vi "myRIO v1.0 Write AO.vi"(7 "Scale Constants Array":T1, 8 "error in (no error)":errorcluster, 9 "dbl Scaled Value List":dbl[](array[numeric]), 10 "Channel List":T5, 11 "myRIO Ref In":T3) -> (0 "error out":errorcluster, 3 "myRIO Ref Out":T3)   [LabVIEW 2021]
uses:
  <vilib>/myRIO/Common/Instrument Driver Framework/myRIO v1.0/AO/typedefs/AO Channels List.ctl
  <vilib>/myRIO/Common/Instrument Driver Framework/myRIO v1.0/AO/typedefs/AO Channels Enum.ctl
  <vilib>/myRIO/Common/Instrument Driver Framework/Utilities/typedefs/myRIO v1.0 Reference.ctl
  <vilib>/myRIO/Common/Instrument Driver Framework/Utilities/typedefs/Generic FPGA Reference.ctl
  <vilib>/myRIO/Common/Instrument Driver Framework/Utilities/typedefs/Analog Scaling Constants List.ctl
  <vilib>/myRIO/Common/Instrument Driver Framework/Utilities/typedefs/Analog Scaling Constants.ctl
  <vilib>/myRIO/Common/Instrument Driver Framework/myRIO v1.0/AO/typedefs/AO Channels FPGA Reference.ctl
  <vilib>/rvi/errors/niLvFpgaAdjustHostInterfaceError.vi
  <vilib>/rvi/interface/nirviReadWriteControl/nirviReadWriteControl.xnode
  <vilib>/rvi/interface/Simulation/niFpgaSimulationCallBeginRW.vi
  NiFpgaLv.dll
panel:
  # "This VI write one analog value to a user specified analog output channel on the myRIO v1.0 hardware. The value is input as a dbl value and scaled to a u16 for input to the FPGA based on the specifications of the DAC. Please see Block Diagram for details."
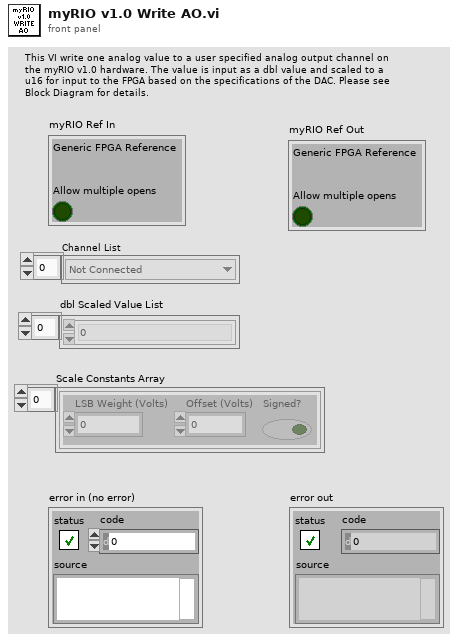
[diagram p1: front panel]
types:
  T1 = typedef "Analog Scaling Constants List.ctl" = T2[]
  T2 = typedef "Analog Scaling Constants.ctl" = cluster{"LSB Weight (Volts)":dbl, "Offset (Volts)":dbl, "Signed?":bool}
  T3 = typedef "myRIO v1.0 Reference.ctl" = cluster{"Generic FPGA Reference":T4, "Allow multiple opens":bool}
  T4 = typedef "Generic FPGA Reference.ctl" = refnum<k20>
  T5 = typedef "AO Channels List.ctl" = T6[]
  T6 = typedef "AO Channels Enum.ctl" = enum16{"Not Connected", "AudioOut/Left", "AudioOut/Right", "C/AO0", "C/AO1", "A/AO0", "A/AO1", "B/AO0", "B/AO1"}
  T7 = typedef "AO Channels FPGA Reference.ctl" = refnum<k20>
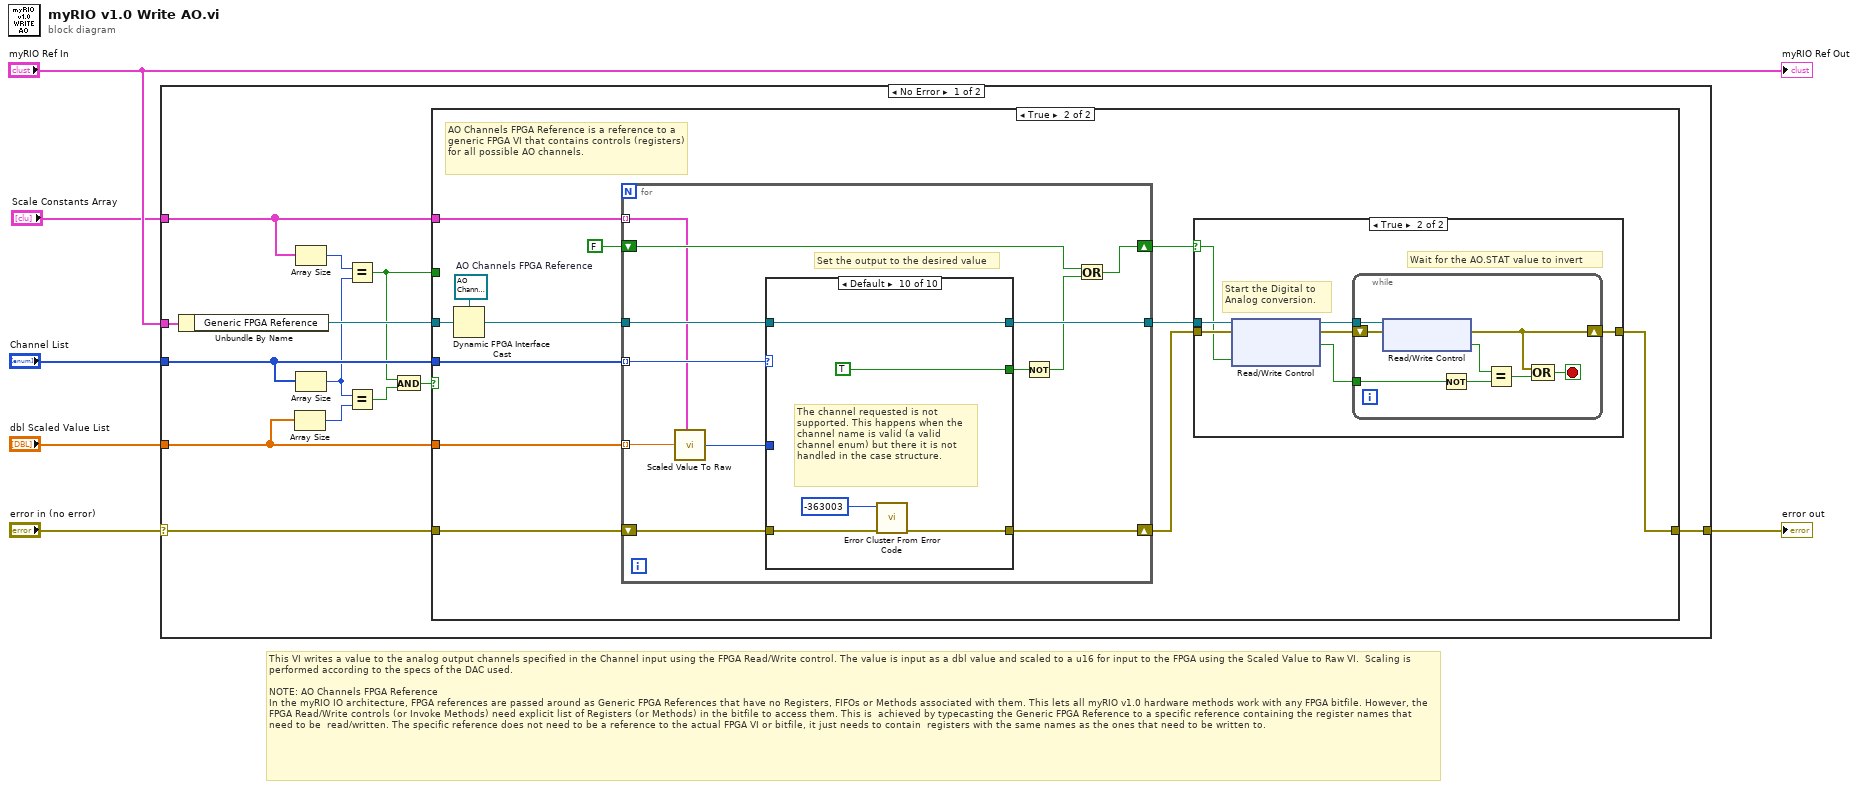
[diagram p0: block diagram]
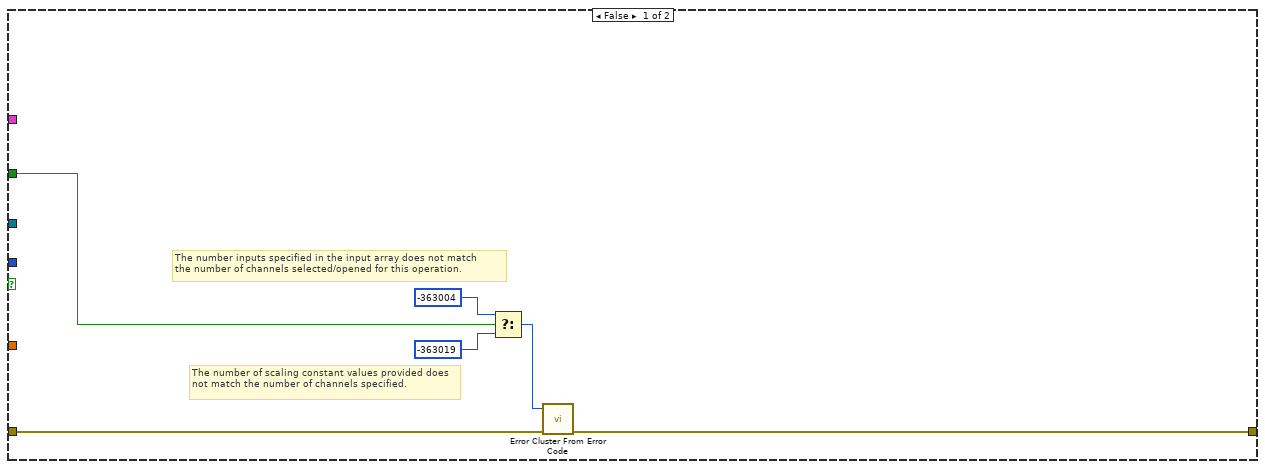
[diagram p2: hidden frame]
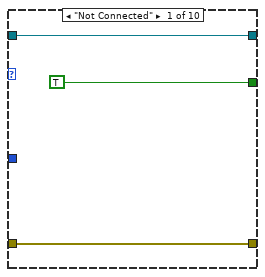
[diagram p4: hidden frame]
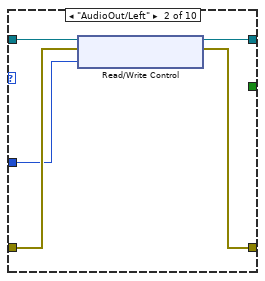
[diagram p5: hidden frame]
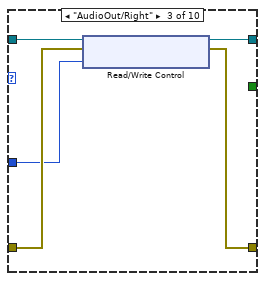
[diagram p6: hidden frame]
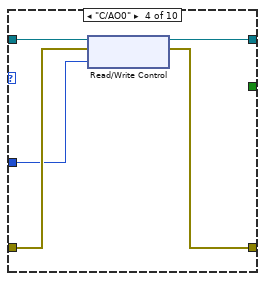
[diagram p7: hidden frame]
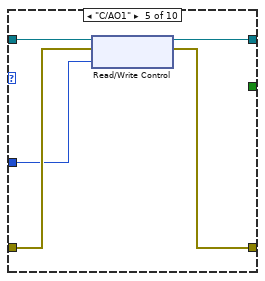
[diagram p8: hidden frame]
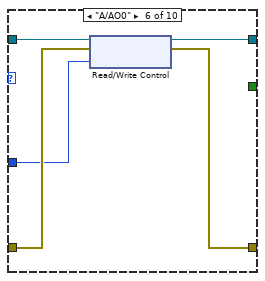
[diagram p9: hidden frame]
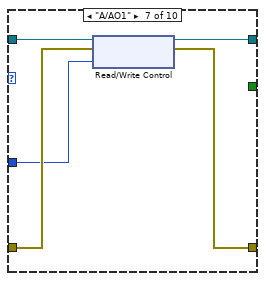
[diagram p10: hidden frame]
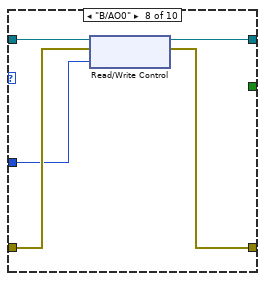
[diagram p11: hidden frame]
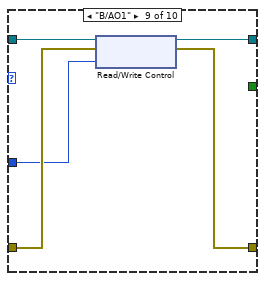
[diagram p12: hidden frame]
diagram:
  # "This VI writes a value to the analog output channels specified in the Channel input using the FPGA Read/Write control. The value is input as a dbl value and scaled to a u16 for input to the FPGA using the Scaled Value to Raw VI.  Scaling is performed according to the specs of the DAC used.\n\nNOTE: AO Channels FPGA Reference\nIn the myRIO IO architecture, FPGA references are passed around as Generic FPGA References that have no Registers, FIFOs or Methods associated with them. This lets all myRIO v1.0 hardware methods work with any FPGA bitfile. However, the  FPGA Read/Write controls (or Invoke Methods) need explicit list of Registers (or Methods) in the bitfile to access them. This is  achieved by typecasting the Generic FPGA Reference to a specific reference containing the register names that need to be  read/written. The specific reference does not need to be a reference to the actual FPGA VI or bitfile, it just needs to contain  registers with the same names as the ones that need to be written to."
  n1 = case shown="No Error" "error in (no error)" {
    selector: "error in (no error)" -> [w15 w114]
    tunnel: [w19 w114] -> w6
    tunnel: "Channel List" -> [w18 _]
    tunnel: "dbl Scaled Value List" -> [w17 _]
    tunnel: "myRIO Ref In" -> [w14 _]
    tunnel: "Scale Constants Array" -> [w12 _]
    frame No Error {
      n2 = Unbundle By Name(w14) -> ("Generic FPGA Reference"=w13:T4)
      n3 = Array Size(array=w17) -> (size(s)=w16:i32)
      n4 = Array Size(array=w12) -> (size(s)=w11:i32)
      n5 = Array Size(array=w18) -> (size(s)=w10:i32)
      n6 = Equal?(x=w11, y=w10) -> (x = y?=w7:bool)
      n7 = Equal?(x=w10, y=w16) -> (x = y?=w9:bool)
      n8 = And(x=w7, y=w9) -> (x .and. y?=w8:bool)
      n9 = case shown="True" w8 {
        tunnel: w15 -> [w25 w35]
        tunnel: w13 -> [_ w32]
        tunnel: [w24 w26] -> w19
        tunnel: w18 -> [_ w34]
        tunnel: w17 -> [_ w33]
        tunnel: w12 -> [_ w27]
        tunnel: w7 -> [w23 _]
        frame False {
          # "The number of scaling constant values provided does not match the number of channels specified."
          # "The number inputs specified in the input array does not match\nthe number of channels selected/opened for this operation."
          n10 = Select(t=-363004 ("error code (0)"), s=w23, f=-363019 ("error code (0)")) -> (s? t:f=w22:i32)
          n11 = call <vilib>:"Error Cluster From Error Code.vi"("error in (no error)"=w25, "error code (0)"=w22) -> ("error out"=w24:errorcluster)  [unwired: 7 in]
        }
        frame True {
          w37 = T7 refnum  # AO Channels FPGA Reference
          # "AO Channels FPGA Reference is a reference to a generic FPGA VI that contains controls (registers) for all possible AO channels."
          n12 = Dynamic FPGA Interface Cast(Session In=w37, Type=w32) -> (Session Out=w36:T7)
          n13 = for {
            tunnel: w36 -> [w65]
            tunnel: w33 -> [w62] mode=indexing
            tunnel: w34 -> [w60] mode=indexing
            shift-right: [w63] -> w30
            shift-left: w35 -> [w64]
            tunnel: [w59] -> w31
            shift-right: [w58] -> w28
            shift-left: FALSE ("AO.GO") -> [w57]
            tunnel: w27 -> [w54] mode=indexing
            # "Set the output to the desired value"
            n14 = call <vilib>:"Scaled Value To Raw.vi"("Scaling Constants"=w54, "dbl Scaled Value"=w62) -> ("u16 Raw Value"=w61:u16)  [unwired: 7 in]
            n15 = case shown="Default" w60 {
              tunnel: w64 -> [w68 w73 w78 w83 w88 w93 w98 w103 w108 w111]
              tunnel: [w68 w72 w77 w82 w87 w92 w97 w102 w107 w112] -> w63
              tunnel: w65 -> [w67 w71 w76 w81 w86 w91 w96 w101 w106 w110]
              tunnel: w61 -> [_ w70 w75 w80 w85 w90 w95 w100 w105 _]
              tunnel: [w67 w69 w74 w79 w84 w89 w94 w99 w104 w110] -> w59
              tunnel: [TRUE ("AO.GO") _ _ _ _ _ _ _ _ TRUE ("AO.GO")] -> w56
              frame "Not Connected" {
              }
              frame "AudioOut/Left" {
                n16 = xnode "Read/Write Control"("FPGA VI Reference In"=w71, "error in"=w73, "AO.AudioOut_L.VAL"=w70) -> ("FPGA VI Reference Out"=w69:T7, "error out"=w72:errorcluster)
              }
              frame "AudioOut/Right" {
                n17 = xnode "Read/Write Control"("FPGA VI Reference In"=w76, "error in"=w78, "AO.AudioOut_R.VAL"=w75) -> ("FPGA VI Reference Out"=w74:T7, "error out"=w77:errorcluster)
              }
              frame "C/AO0" {
                n18 = xnode "Read/Write Control"("FPGA VI Reference In"=w81, "error in"=w83, "AO.C_0.VAL"=w80) -> ("FPGA VI Reference Out"=w79:T7, "error out"=w82:errorcluster)
              }
              frame "C/AO1" {
                n19 = xnode "Read/Write Control"("FPGA VI Reference In"=w86, "error in"=w88, "AO.C_1.VAL"=w85) -> ("FPGA VI Reference Out"=w84:T7, "error out"=w87:errorcluster)
              }
              frame "A/AO0" {
                n20 = xnode "Read/Write Control"("FPGA VI Reference In"=w91, "error in"=w93, "AO.A_0.VAL"=w90) -> ("FPGA VI Reference Out"=w89:T7, "error out"=w92:errorcluster)
              }
              frame "A/AO1" {
                n21 = xnode "Read/Write Control"("FPGA VI Reference In"=w96, "error in"=w98, "AO.A_1.VAL"=w95) -> ("FPGA VI Reference Out"=w94:T7, "error out"=w97:errorcluster)
              }
              frame "B/AO0" {
                n22 = xnode "Read/Write Control"("FPGA VI Reference In"=w101, "error in"=w103, "AO.B_0.VAL"=w100) -> ("FPGA VI Reference Out"=w99:T7, "error out"=w102:errorcluster)
              }
              frame "B/AO1" {
                n23 = xnode "Read/Write Control"("FPGA VI Reference In"=w106, "error in"=w108, "AO.B_1.VAL"=w105) -> ("FPGA VI Reference Out"=w104:T7, "error out"=w107:errorcluster)
              }
              frame Default {
                # "The channel requested is not supported. This happens when the channel name is valid (a valid channel enum) but there it is not handled in the case structure."
                n24 = call <vilib>:"Error Cluster From Error Code.vi"("error in (no error)"=w111, "error code (0)"=-363003) -> ("error out"=w112:errorcluster)  [unwired: 7 in]
              }
            }
            n25 = Not(x=w56) -> (.not. x?=w55:bool)
            n26 = Or(x=w57, y=w55) -> (x .or. y?=w58:bool)
          }
          n27 = case shown="True" w28 {
            selector: w28 -> [_ w43]
            tunnel: w31 -> [_ w45]
            tunnel: w30 -> [w38 w44]
            tunnel: [w38 w39] -> w26
            frame False {
            }
            frame True {
              # "Wait for the AO.STAT value to invert"
              # "Start the Digital to Analog conversion."
              n28 = xnode "Read/Write Control"("FPGA VI Reference In"=w45, "error in"=w44, "AO.SYS.GO"=w43) -> ("FPGA VI Reference Out"=w41:T7, "error out"=w40:errorcluster, "AO.SYS.STAT"=w42:bool)
              n29 = while {
                tunnel: w42 -> [w50]
                tunnel: w41 -> [w52]
                shift-right: [w47] -> w39
                shift-left: w40 -> [w53]
                stop <- w48 stop-if-true
                n30 = xnode "Read/Write Control"("FPGA VI Reference In"=w52, "error in"=w53) -> ("error out"=w47:errorcluster, "AO.SYS.STAT"=w51:bool)  [unwired: 1 out]
                n31 = Not(x=w50) -> (.not. x?=w49:bool)
                n32 = Equal?(x=w51, y=w49) -> (x = y?=w46:bool)
                n33 = Compound Arithmetic op=OR(w47, w46) -> (w48:bool)
              }
            }
          }
        }
      }
    }
    frame Error {
      # "There is an incoming error so there is nothing to do."
    }
  }
  "error out" <- w6
  "myRIO Ref Out" <- "myRIO Ref In"
